vi "Register HTTP Services.vi"(8 "error in (no error)":errorcluster, 11 "SOL-Server in":refnum<class "SOL-Server.lvclass">) -> (0 "error out":errorcluster, 3 "SOL-Server out":refnum<class "SOL-Server.lvclass">)   [LabVIEW 2020, in "Summer of LabVIEW.lvlib" / "SOL-Server.lvclass"]
uses:
  SOL-Server.lvclass
  SOL-Server.lvclass/SOL-Server.ctl
  <vilib>/IlluminatedG/IG HTTP Server/HTTP Server/Server/Server.lvclass
  Challenge DB/Challenge DB.lvclass
  C:/dev/IlluminatedG/lv-sol-22/Challenge DB/Challenge DB.lvclass
  C:/Program Files (x86)/National Instruments/LabVIEW 2020/vi.lib/IlluminatedG/IG HTTP Server/HTTP Server/Service/Service.lvclass
  Submission DB/Submission DB.lvclass
  C:/dev/IlluminatedG/lv-sol-22/Submission DB/Submission DB.lvclass
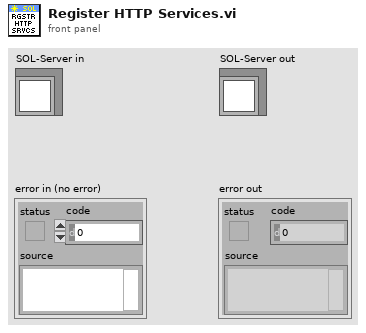
[diagram p1: front panel]
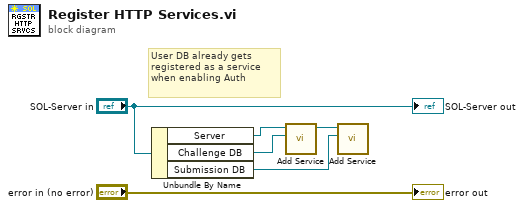
[diagram p0: block diagram]
diagram:
  # "User DB already gets registered as a service when enabling Auth"
  n1 = Unbundle By Name("SOL-Server in") -> ("Server"=w5:refnum<class "Server.lvclass">, "Challenge DB"=w4:refnum<class "Challenge DB.lvclass">, "Submission DB"=w2:refnum<class "Submission DB.lvclass">)
  n2 = call <vilib>:"Add Service.vi"("Service"=w4, "Server in"=w5) -> ("Server out"=w3:refnum<class "Server.lvclass">)  [unwired: 8 in, 1 out]
  n3 = call <vilib>:"Add Service.vi"("Service"=w2, "Server in"=w3) -> ()  [unwired: 8 in, 2 out]
  "error out" <- "error in (no error)"
  "SOL-Server out" <- "SOL-Server in"
